vi "JSON Tree to ChannelList.vi"(8 "error in (no error)":errorcluster, 11 "JSON Tree Out":variant) -> (0 "error out":errorcluster, 2 "ChannelList":T1, 3 "JSON Tree Out Passthrough":variant)   [LabVIEW 2015, in "SLSC Switch.lvlib" / "SLSC Switch.lvclass"]
uses:
  SLSC Switch.lvclass
  Controls/JSON.ChannelList.ctl
  <vilib>/LVH/i3 JSON/JSON Parsing/Get Object Parameter Files/Get Object Parameter - Object.vi
  <vilib>/LVH/i3 JSON/i3-json.lvlib
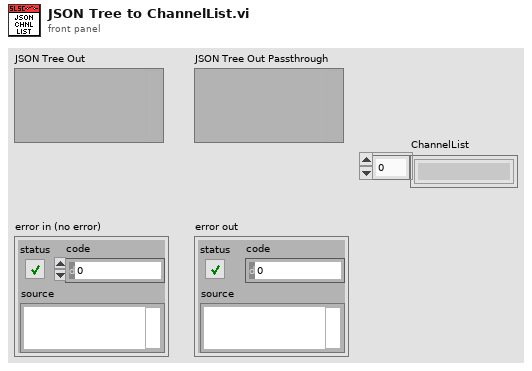
[diagram p1: front panel]
types:
  T1 = typedef "SLSC Switch.lvlib/SLSC Switch.lvclass/JSON.ChannelList.ctl" = string[]
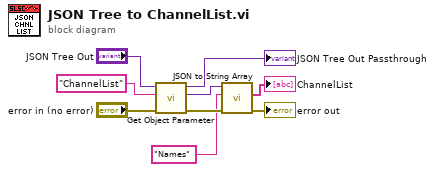
[diagram p0: block diagram]
diagram:
  n1 = call-poly <vilib>:"Get Object Parameter.vi"("error in (no error)"="error in (no error)", "Parameter Name"="ChannelList", "JSON Tree In (JSON Object)"="JSON Tree Out") -> ("error out"=w8:errorcluster, "JSON Object"=w5:variant, "JSON Tree Out Passthrough"=→"JSON Tree Out Passthrough":variant)  [unwired: 5 in, 1 out]
  n2 = call "JSON to String Array.vi"("error in (no error)"=w8, "Parameter Name"="Names", "JSON Tree In"=w5) -> ("error out"=→"error out":errorcluster, "Array"=→"ChannelList":string[])  [unwired: 6 in, 1 out]
